vi "RT Main.vi"() -> ()   [LabVIEW 2013]
uses:
  Web Messaging Palette/Web Messaging API.lvlib
panel:
  in  "stop":bool
  out "myRIO LEDs":bool[](array[boolean])
  in  "Run Test":bool
  out "error out":errorcluster
  in  "Services Token":string
  # "This app demonstrates how to use Web Messaging for NI myRIO\n-Get started by visiting https://myrio.niwsc.com and creating an account\n-On the myRIO Web App click 'My account' and then click 'Services token'\n-On the Services token tab click 'Generate new token'\n-Install the HTTP Client with SSL Support onto the myRIO\n-Configure the myRIO to connect to WiFi with internet access\n-Copy your new services token and paste it in this VI's Services Token control\n-Run the RT Main.vi on the myRIO\n-Run this VI and see the messages and errors from the myRIO"
  # "If you deploy this VI to run as startup, make sure to set the Services Token to default to your services token or load your Services Token from a file or string constant."
  # "An LED lights up each time an \nerror message is sent to the \nWeb Messaging service"
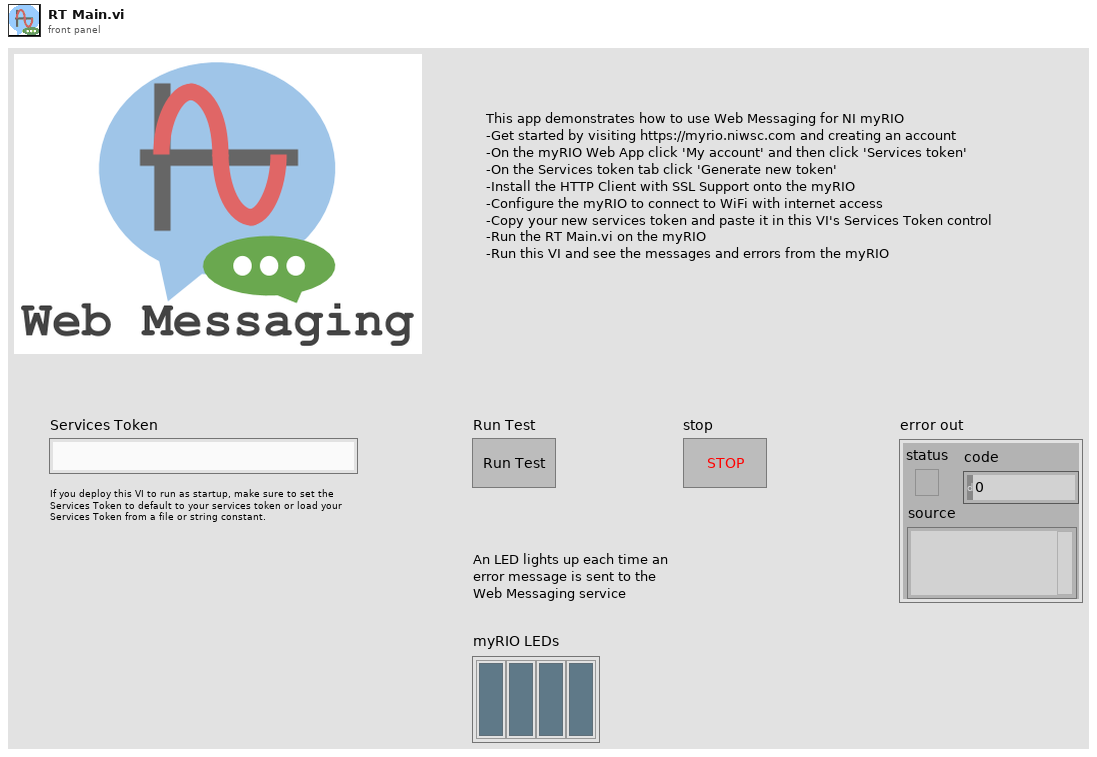
[diagram p1: front panel]
types:
  T1 = typedef "Web Messaging API.lvlib/Web Messaging Handle.ctl" = cluster{"Services token":string}
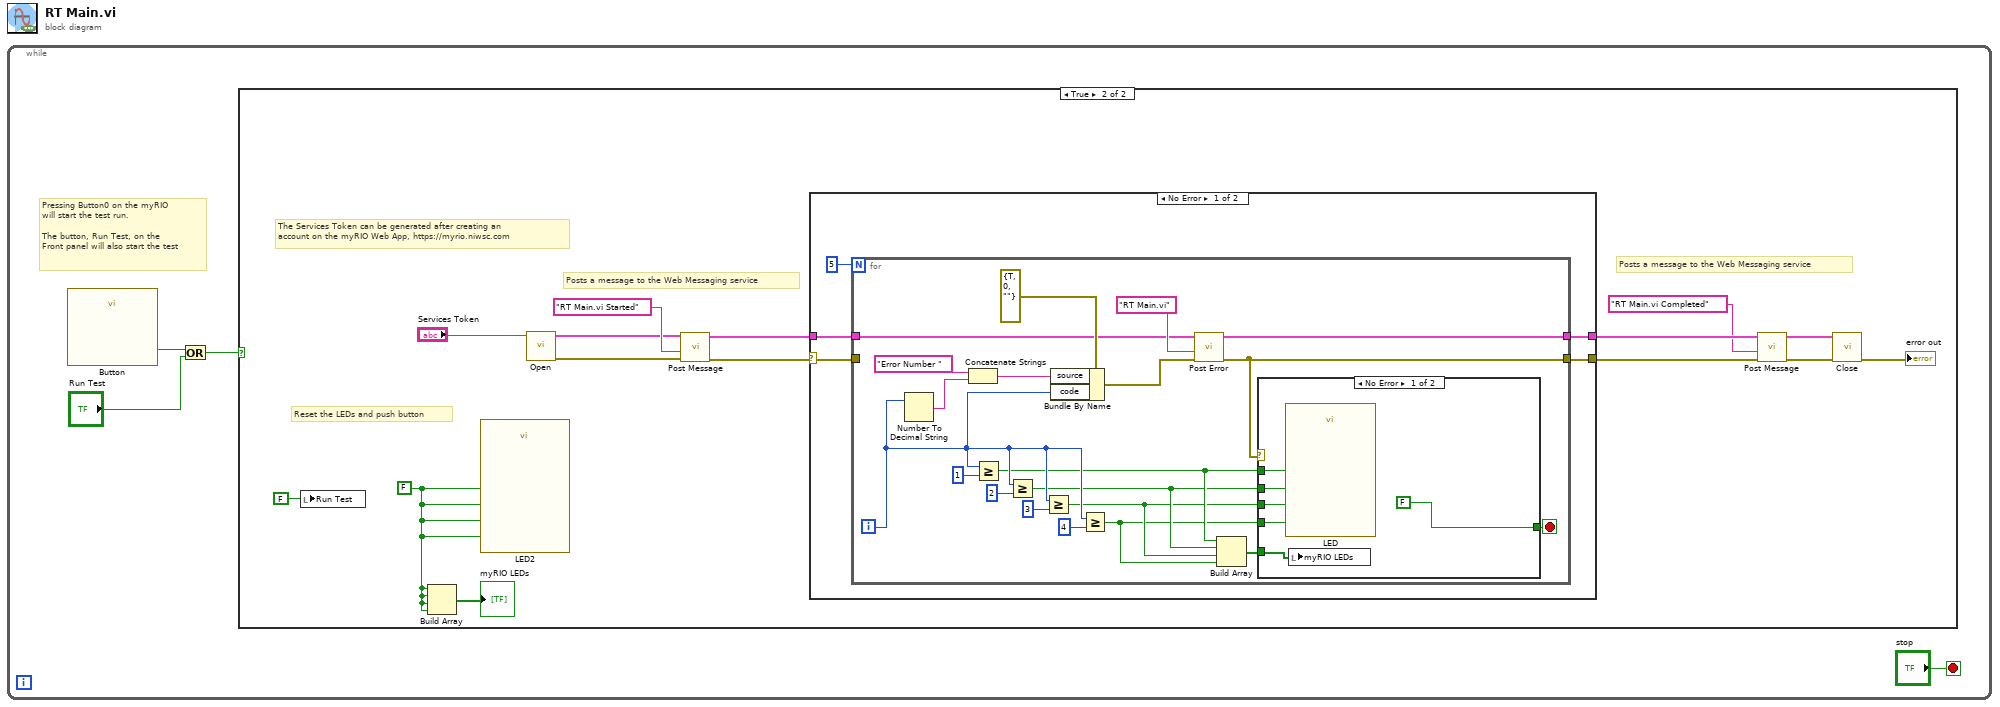
[diagram p0: block diagram]
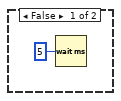
[diagram p2: hidden frame]
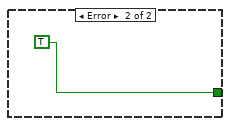
[diagram p3: hidden frame]
diagram:
  n1 = while {
    stop <- "stop" stop-if-true
    # "Pressing Button0 on the myRIO \nwill start the test run.\n\nThe button, Run Test, on the\nFront panel will also start the test"
    n2 = call "Button"() -> ("Value"=w4:bool)  [unwired: 26 in, 1 out]
    n3 = Or(x=w4, y="Run Test") -> (x .or. y?=w2:bool)
    n4 = case shown="True" w2 {
      frame False {
        n5 = Wait (ms)(milliseconds to wait=u32 5) -> ()  [unwired: 1 out]
      }
      frame True {
        w10 = FALSE ("Error 1")
        # "Reset the LEDs and push button"
        # "Posts a message to the Web Messaging service"
        # "Posts a message to the Web Messaging service"
        # "The Services Token can be generated after creating an \naccount on the myRIO Web App, https://myrio.niwsc.com"
        n6 = local write "Run Test"(FALSE ("Value")) -> ()
        n7 = Build Array(w10, w10, w10, w10) -> (→"myRIO LEDs":bool[])
        n8 = call "LED2"("Error 1"=w10, "Error 2"=w10, "Error 3"=w10, "Error 4"=w10) -> ()  [unwired: 23 in, 1 out]
        n9 = call "Open.vi"("Services Token"="Services Token") -> ("error out"=w8:errorcluster, "Web App Handle"=w7:T1)  [unwired: 9 in]
        n10 = call "Post Message.vi"("error in"=w8, "message"="RT Main.vi Started", "Web App Handle In"=w7) -> ("error out"=w19:errorcluster, "Web App Handle Out"=w18:T1)  [unwired: 6 in, 1 out]
        n11 = case shown="No Error" w19 {
          selector: w19 -> [w22 w54]
          tunnel: [w21 w54] -> w20
          tunnel: w18 -> [w24 w53]
          tunnel: [w23 w53] -> w17
          frame No Error {
            n12 = for {
              N: 5 -> [_]
              tunnel: w24 -> [w28]
              tunnel: [w26] -> w23
              tunnel: w22 -> [_]
              tunnel: [w27] -> w21
              i -> [w37]
              stop <- w36 stop-if-true
              n13 = Number To Decimal String(number=w37) -> (decimal integer string=w43:string)  [unwired: 1 in]
              n14 = Concatenate Strings("Error Number " ("string"), w43) -> (w42:string)
              n15 = Greater Or Equal?(x=w37, y=1) -> (x >= y?=w35:bool)
              n16 = Greater Or Equal?(x=w37, y=2) -> (x >= y?=w34:bool)
              n17 = Greater Or Equal?(x=w37, y=3) -> (x >= y?=w33:bool)
              n18 = Bundle By Name(cluster=errorcluster {"status"=TRUE, "code"=0, "source"=""} ("error IO"), "source"=w42, "code"=w37) -> (w30:errorcluster)
              n19 = Greater Or Equal?(x=w37, y=4) -> (x >= y?=w32:bool)
              n20 = call "Post Error.vi"("Web App Handle In"=w28, "message"="RT Main.vi", "error in"=w30) -> ("Web App Handle Out"=w26:T1, "error out"=w27:errorcluster)  [unwired: 5 in, 1 out]
              n21 = Build Array(w35, w34, w33, w32) -> (w31:bool[])
              n22 = case shown="No Error" w27 {
                tunnel: w35 -> [w51 _]
                tunnel: w34 -> [w50 _]
                tunnel: w33 -> [w49 _]
                tunnel: w32 -> [w48 _]
                tunnel: [FALSE TRUE] -> w36
                tunnel: w31 -> [w46 _]
                frame No Error {
                  n23 = call "LED"("Error 1"=w51, "Error 2"=w50, "Error 3"=w49, "Error 4"=w48) -> ()  [unwired: 23 in, 1 out]
                  n24 = local write "myRIO LEDs"(w46) -> ()
                }
                frame Error {
                }
              }
            }
          }
          frame Error {
          }
        }
        n25 = call "Post Message.vi"("error in"=w20, "message"="RT Main.vi Completed", "Web App Handle In"=w17) -> ("error out"=w13:errorcluster, "Web App Handle Out"=w12:T1)  [unwired: 6 in, 1 out]
        n26 = call "Close.vi"("error in"=w13, "Web App Handle"=w12) -> ("error out"=→"error out":errorcluster)  [unwired: 9 in]
      }
    }
  }
